vi "Control_DAQ_USB6008.vi"(8 "Error input":errorcluster, 10 "Data written to digital output channels":bool[](array[boolean]), 11 "Digital output ports":tag="Dev1/port0/line0:5") -> (0 "Error output":errorcluster)   [LabVIEW 2017]
uses:
  <vilib>/DAQmx/write.llb/DAQmx Write (Digital 1D Bool 1Chan 1Samp).vi
  <vilib>/DAQmx/create/channels.llb/DAQmx Create Channel (DO-Digital Output).vi
  <vilib>/DAQmx/miscellaneous.llb/DAQmx Fill In Error Info.vi
panel:
  out "Status":string
  # "Control USB6008 DAQ device"
  # "Additional info:\n1. USB6008 PO.0&PO.1: Dev1/port0/line0:1\n        Dev1: Device connected to test pc\n        port0: Port of USB6008\n        Line0:1: Selects PO.0 & PO.1 for communication\n\n2. Active Low and Active High\n         Active Low: 0 enables the e-stop/Palm Button \n         Active High: 1 disables the e-stop/Palm Button"
  # "P0.4"
  # "P0.5"
  # "P0.7"
  # "P0.3"
  # "P0.6"
  # "P0.1"
  # "P0.2"
  # "P0.0"
  # "J805-1"
  # "J805-4"
  # "J805-9"
  # "J805-14"
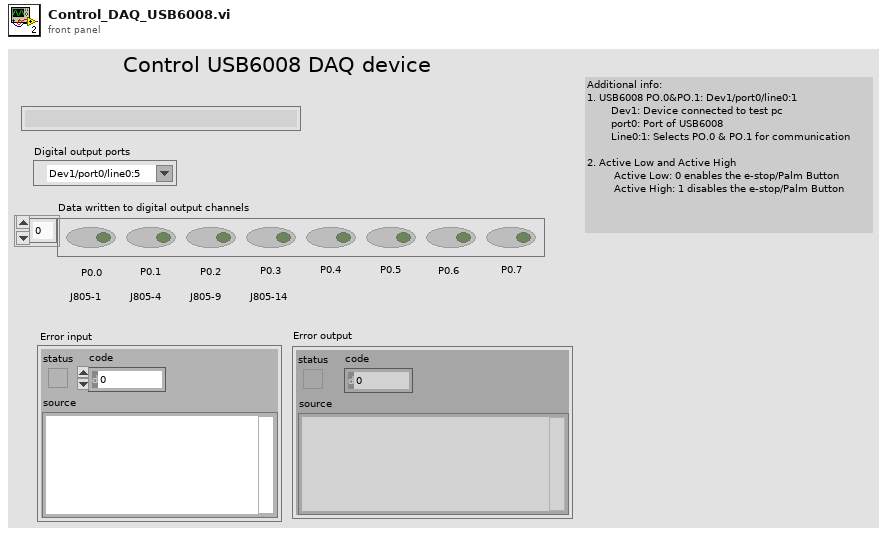
[diagram p1: front panel]
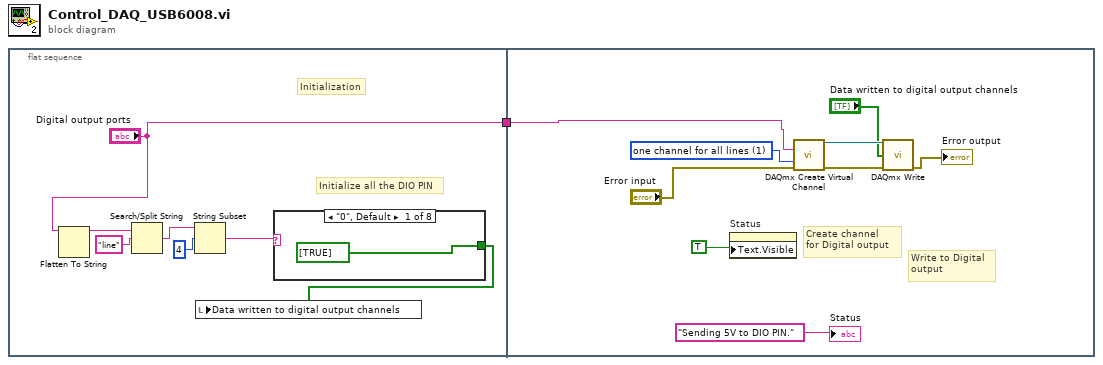
[diagram p0: block diagram]
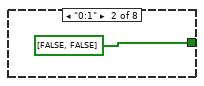
[diagram p2: hidden frame]
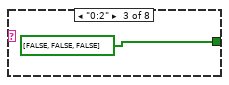
[diagram p3: hidden frame]
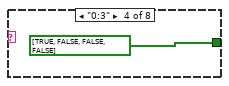
[diagram p4: hidden frame]
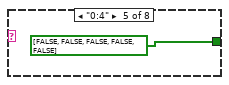
[diagram p5: hidden frame]
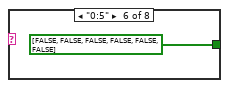
[diagram p6: hidden frame]
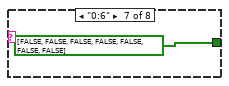
[diagram p7: hidden frame]
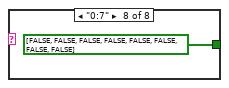
[diagram p8: hidden frame]
diagram:
  n1 = flat-sequence {
    tunnel: ["Digital output ports"] -> w1
    tunnel: w1 -> [w25]
    frame #0 {
      # "Initialize all the DIO PIN"
      # "Initialization"
      n2 = Flatten To String(anything="Digital output ports") -> (data string=w5:string)  [unwired: 3 in, 2 out]
      n3 = Search/Split String(string=w5, search string/char (-)="line") -> (match + rest of string=w6:string)  [unwired: 1 in, 2 out]
      n4 = String Subset(string=w6, offset (0)=4) -> (substring=w7:string)  [unwired: 1 in]
      n5 = case shown="\"0\", Default" w7 {
        tunnel: [bool[] [TRUE] ("Data written to digital output channels") bool[] [FALSE, FALSE] ("Data written to digital output channels") bool[] [FALSE, FALSE, FALSE] ("Data written to digital output channels") bool[] [TRUE, FALSE, FALSE, FALSE] ("Data written to digital output channels") bool[] [FALSE, FALSE, FALSE, FALSE, FALSE] ("Data written to digital output channels") bool[] [FALSE, FALSE, FALSE, FALSE, FALSE, FALSE] ("Data written to digital output channels") bool[] [FALSE, FALSE, FALSE, FALSE, FALSE, FALSE, FALSE] ("Data written to digital output channels") bool[] [FALSE, FALSE, FALSE, FALSE, FALSE, FALSE, FALSE, FALSE] ("Data written to digital output channels")] -> w8
        frame "0", Default {
        }
        frame "0:1" {
        }
        frame "0:2" {
        }
        frame "0:3" {
        }
        frame "0:4" {
        }
        frame "0:5" {
        }
        frame "0:6" {
        }
        frame "0:7" {
        }
      }
      n6 = local write "Data written to digital output channels"(w8) -> ()
    }
    frame #1 {
      w20 = 1 items=["one channel for each line", "one channel for all lines"] ("line grouping")
      # "Write to Digital \noutput"
      # "Create channel \nfor Digital output"
      n7 = property on="Status" class="Str"("Text.Visible"=TRUE) -> ()  [unwired: 2 in, 2 out]
      n8 = call-poly <vilib>:"DAQmx Create Virtual Channel.vi"("lines"=w25, "line grouping"=w20, "error in"="Error input") -> ("task out"=w22:refnum<k21>, "error out"=w21:errorcluster)  [unwired: 11 in]
      n9 = call-poly <vilib>:"DAQmx Write.vi"("task/channels in"=w22, "data"="Data written to digital output channels", "error in"=w21) -> ("error out"=→"Error output":errorcluster)  [unwired: 10 in, 2 out]
      "Status" <- "Sending 5V to DIO PIN." ("Status")
    }
  }
